vi "Thingworx_Write_image.vi"(9 "image data":T1, 11 "Thingworx":string(xcontrol)) -> ()   [LabVIEW 2020]
uses:
  TW_XControl.xctl
  <vilib>/picture/picture.llb/imagedata.ctl
panel:
  out "Image":picture
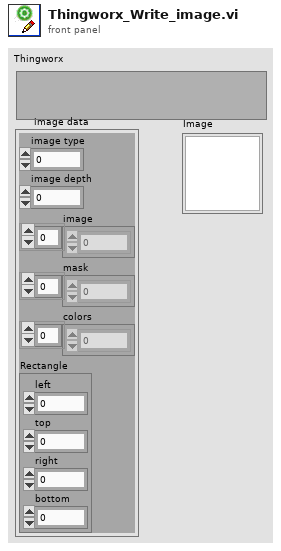
[diagram p1: front panel]
types:
  T1 = typedef "imagedata.ctl" = cluster{"image type":i32, "image depth":i32, "image":u8[], "mask":u8[], "colors":u32[], "Rectangle":cluster{"left":i16, "top":i16, "right":i16, "bottom":i16}}
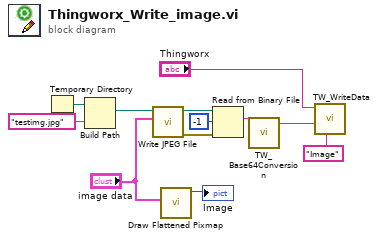
[diagram p0: block diagram]
diagram:
  n1 = Temporary Directory() -> (w3:path)
  n2 = Build Path(base path=w3, name or relative path="testimg.jpg") -> (appended path=w1:path)
  n3 = call <vilib>:"Write JPEG File.vi"("image data"="image data", "path to JPEG file"=w1) -> ("error out"=w8:errorcluster, "path"=w7:path)  [unwired: 8 in]
  n4 = call <vilib>:"Draw Flattened Pixmap.vi"("image data"="image data") -> ("new picture"=→"Image":picture)  [unwired: 8 in]
  n5 = Read from Binary File(8:w8, 10:-1 ("count (1)"), 11:w7) -> (2:w6:string)  [unwired: 3 in, 3 out]
  n6 = call "TW_Base64Conversion.vi"("String"=w6) -> ("Base64 String"=w5:string)  [unwired: 8 in, 2 out]
  n7 = call "TW_WriteData.vi"("Type"="Image", "value"=w5, "Property"="Thingworx") -> ()  [unwired: 9 in]
